vi "Read Observer Refs.vi"(8 "error in (no error)":errorcluster, 11 "Data Subject in":refnum<class "Publisher.lvclass">) -> (0 "error out":errorcluster, 2 "Observer Refs":refnum<queue>[](array[refnum]), 3 "Data Subject out":refnum<class "Publisher.lvclass">)   [LabVIEW 2014, in "Publisher.lvclass"]
uses:
  Publisher.lvclass
  Data/Data.lvclass
  Publisher.lvclass/Publisher.ctl
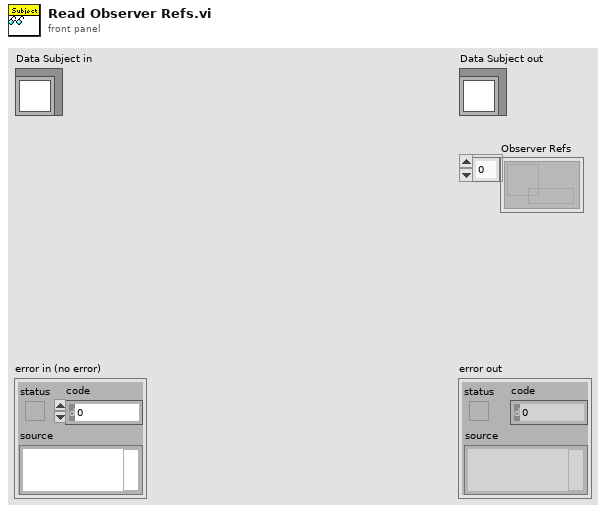
[diagram p1: front panel]
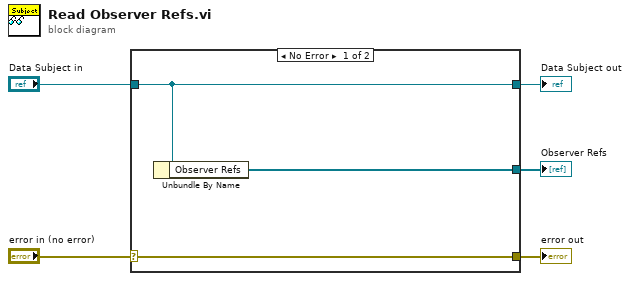
[diagram p0: block diagram]
diagram:
  n1 = case shown="No Error" "error in (no error)" {
    selector: "error in (no error)" -> [w8 w9]
    tunnel: [w8 w9] -> w4
    tunnel: [w7 w10] -> w2
    tunnel: "Data Subject in" -> [w7 w10]
    tunnel: [w6 _] -> w1
    frame No Error {
      n2 = Unbundle By Name(w7) -> ("Observer Refs"=w6:refnum<queue>[])
    }
    frame Error {
    }
  }
  "error out" <- w4
  "Data Subject out" <- w2
  "Observer Refs" <- w1
